vi "SNMP Build OID.vi"(0 "OID String":string) -> (1 "OID Length":u8[](array[numeric]), 2 "OID Byte Array":u8[](array[numeric]) format="%.0x")   [LabVIEW 2017]
doc: "This VI converts a string OID to a byte array. It requires a string representing the OID as input and provides the length of the OID and the OID as a byte array as output."
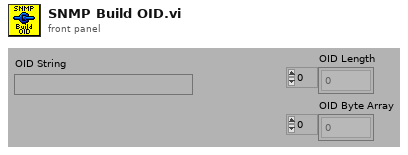
[diagram p1: front panel]
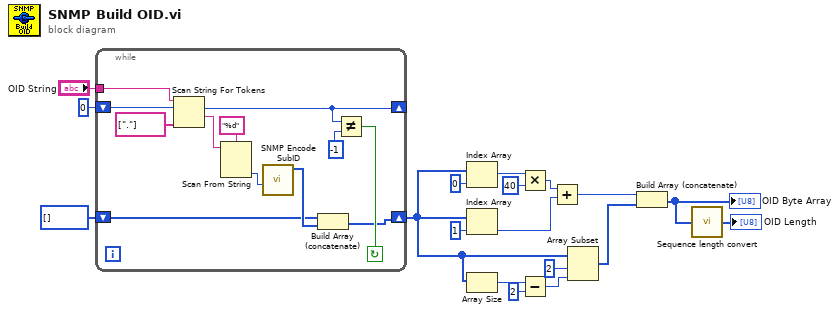
[diagram p0: block diagram]
diagram:
  n1 = while {
    shift-left: u8[] [] -> [w20]
    shift-right: [w19] -> w8
    shift-left: 0 ("offset past token") -> [w29]
    shift-right: [w28] -> _
    tunnel: "OID String" -> [w26]
    stop <- w27 continue-if-true
    n2 = Scan String For Tokens(6:string[] ["."] ("delimiters (\\s,\\t,\\r,\\n)"), 8:w29, 9:w26) -> (1:w24:string, 2:w28:i32)  [unwired: 5 out]
    n3 = Scan From String(format string="%d", input string=w24) -> (output 1=w22:i32)  [unwired: 2 in, 4 out]
    n4 = call "SNMP Encode SubID.vi"("SubID String"=w22) -> ("SubID byte array"=w21:u8[])  [unwired: 9 out]
    n5 = Build Array (concatenate)(w20, w21) -> (w19:u8[])
    n6 = Not Equal?(x=w28, y=-1) -> (x != y?=w27:bool)
  }
  n7 = Index Array(array=w8, index=0) -> (element=w13:u8)
  n8 = Index Array(array=w8, index=1) -> (element=w10:u8)
  n9 = Array Size(array=w8) -> (size(s)=w7:i32)
  n10 = Multiply(x=w13, y=u8 40) -> (x*y=w11:u8)
  n11 = Subtract(x=w7, y=2) -> (x-y=w6:i32)
  n12 = Add(x=w11, y=w10) -> (x+y=w3:u8)
  n13 = Array Subset(array=w8, index=2, length=w6) -> (w4:u8[])
  n14 = Build Array (concatenate)(w3, w4) -> (w2:u8[])
  "OID Byte Array" <- w2
  n15 = call "Sequence length convert.vi"("Sequence"=w2) -> ("Sequence Length"=→"OID Length":u8[])  [unwired: 4 out]
